vi "Read Paths.vi"(0 "Path Group in":refnum<class "Path Group.lvclass">, 11 "error in":errorcluster) -> (4 "Path Group out":refnum<class "Path Group.lvclass">, 6 "Paths":refnum<class "Path.lvclass">[](array[class]), 15 "error out":errorcluster)   [LabVIEW 2023, in "RFFixtureCharact.Public.lvlib"]
uses:
  RFFixtureCharact.Public.lvlib
  Common/Base Classes/Path Group/Path Group.lvclass
  Common/Base Classes/Path/Path.lvclass
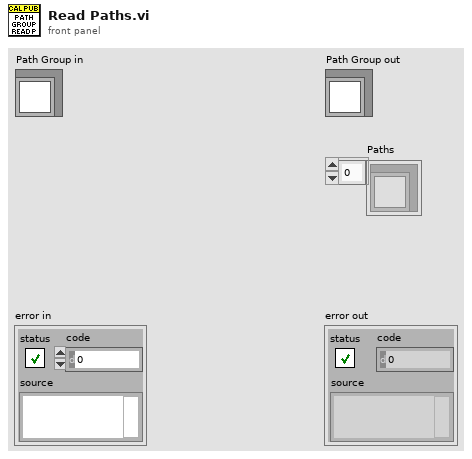
[diagram p1: front panel]
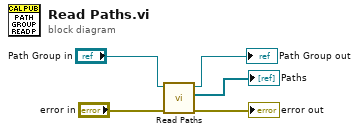
[diagram p0: block diagram]
diagram:
  n1 = call-dynamic "Read Paths.vi"("error in (no error)"="error in", "Cable Path Group in"="Path Group in") -> ("error out"=→"error out":errorcluster, "Paths"=→"Paths":refnum<class "Path.lvclass">[], "Cable Path Group out"=→"Path Group out":refnum<class "Path Group.lvclass">)  [unwired: 7 in]
